vi "PelletronQuery.vi"() -> ()   [LabVIEW 2012]
uses:
  <vilib>/Utility/miscctls.llb/LVPointTypeDef.ctl
  <vilib>/addons/database/Auxilliary.llb/DB Tools Cursor Type.ctl
  <userlib>/_OpenG.lib/array/array.llb/Index 1D Array Elements (String)__ogtk.vi
  <vilib>/addons/database/Connection.llb/Conn Execute.vi
  <vilib>/addons/database/Recordset.llb/Rec Fetch Recordset Data (R).vi
  <vilib>/addons/database/Recordset.llb/Rec Destroy - Connection.vi
  <vilib>/Utility/file.llb/Write To Spreadsheet File (string).vi
  <vilib>/addons/database/_DB Variant To Data/Database Variant To Data.xnode
  <vilib>/addons/database/NI_Database_API.lvlib
panel:
  in  "stop":bool
  in  "Tab Control":T1(tab)
  in  "Active Y Scale":u16(ring) items=["Voltage (MV)", "Current (µA)", "Voltage (kV)", "Pressure (torr)", "Radiation (mr/hr)"]
  in  "X Maximum":dbl format="%<%I:%M:%S %p\n%m/%d/%Y>T"
  in  "X Autoscale":bool=TRUE
  in  "X Minimum":dbl format="%<%I:%M:%S %p\n%m/%d/%Y>T"
  in  "Y Autoscale":bool=TRUE
  in  "Y Maximum":dbl
  in  "Y Minimum":dbl
  in  "Plot":bool
  in  "Limits":T2={"Lower Timestamp Range"=timestamp(0 s since 1904-01-01), "Upper Timestamp Range"=timestamp(0 s since 1904-01-01), "Lower High Voltage"=0.0, "Higher High Voltage"=inf, "Lower Power Supply"=0.0, "Higher Power Supply"=inf}
  in  "Independent Variable":enum32{"Time", "ID"}(radio)
  in  "Pelletron Properties":i32[](listbox)
  out "XY Graph":cluster{ext[], dbl[]}[](graph)
  in  "Write":bool
  in  "Pull Data":bool
  in  "Limits 2":T2
  out "Pelletron Data":string[][](table)
  in  "Save Path":path=path "C:/Users/Clavius/Desktop/Database Query files/New_Pelletron_Query.csv"
  out "error out":errorcluster
  in  "Clear Errors?":bool
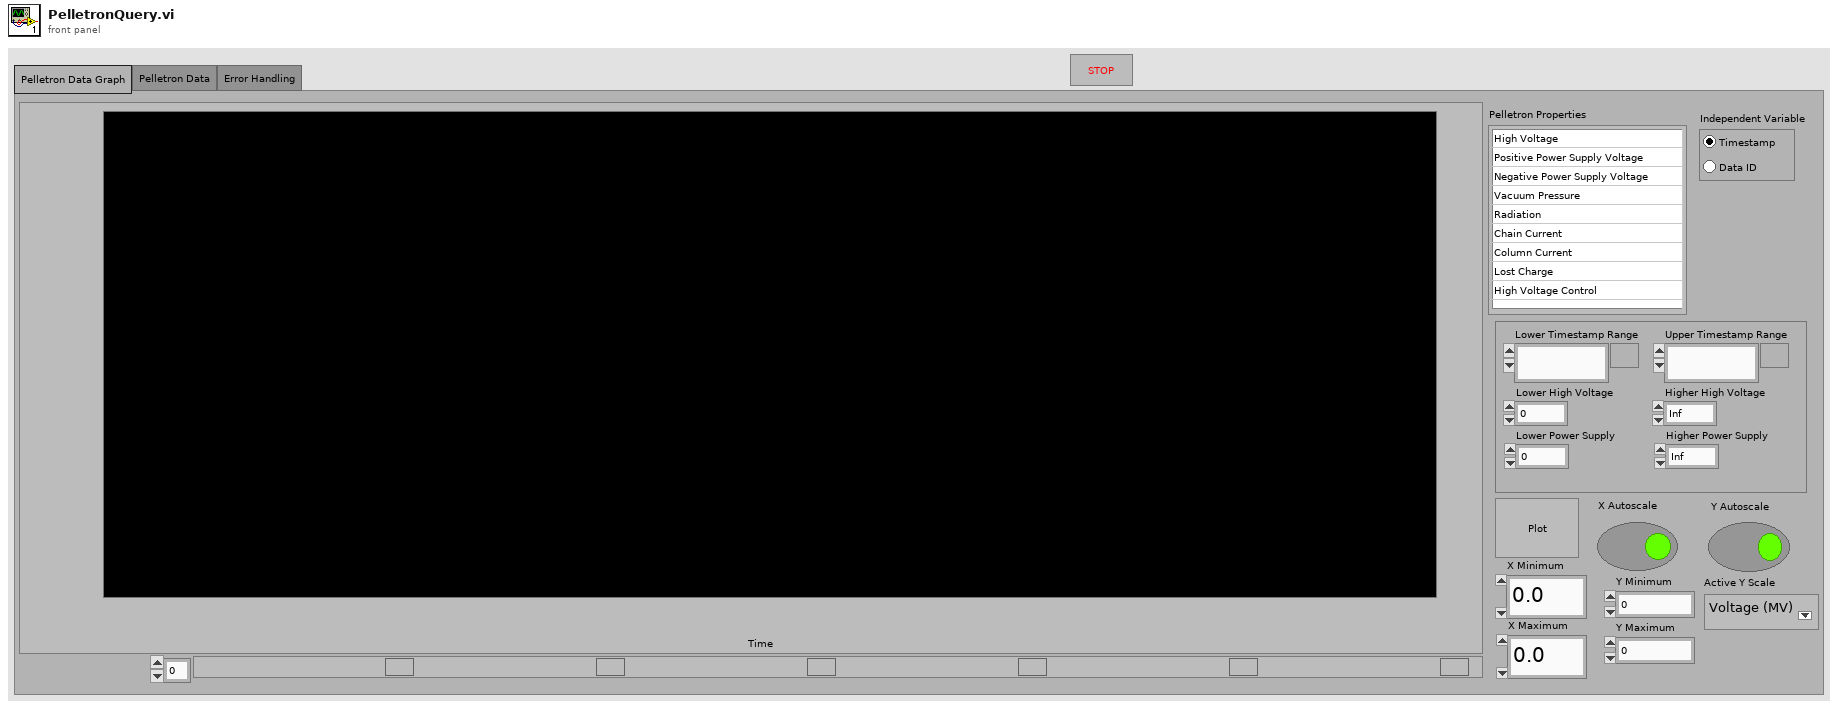
[diagram p1: front panel]
types:
  T1 = enum32{"Pelletron Data Graph", "Pelletron Data", "Error Handling"}
  T2 = cluster{"Lower Timestamp Range":timestamp, "Upper Timestamp Range":timestamp, "Lower High Voltage":dbl, "Higher High Voltage":dbl, "Lower Power Supply":dbl, "Higher Power Supply":dbl}
  T3 = typedef "LVPointTypeDef.ctl" = cluster{"Horizontal":i16, "Vertical":i16}
  T4 = typedef "NI_Database_API.lvlib/DB Tools Cursor Type.ctl" = enum16{"forward-only", "keyset", "dynamic", "static"}
  T5 = cluster{"Pelletron ID":i32[], "Integer Timestamp":dbl[], "High Voltage":dbl[], "Positive High Voltage Supply":dbl[], "Negative High Voltage Supply":dbl[], "Vaccuum Pressure":dbl[], "Radiation":dbl[], "Chain Current":dbl[], "Column Current":dbl[], "Lost Charge":dbl[], "High Voltage Control":dbl[], "Control Difference":dbl[]}
  T6 = typedef "NI_Database_API.lvlib/Conn ObjectReference.ctl" = refnum<k1>
  T7 = typedef "NI_Database_API.lvlib/Rec ObjectReference.ctl" = refnum<k1>
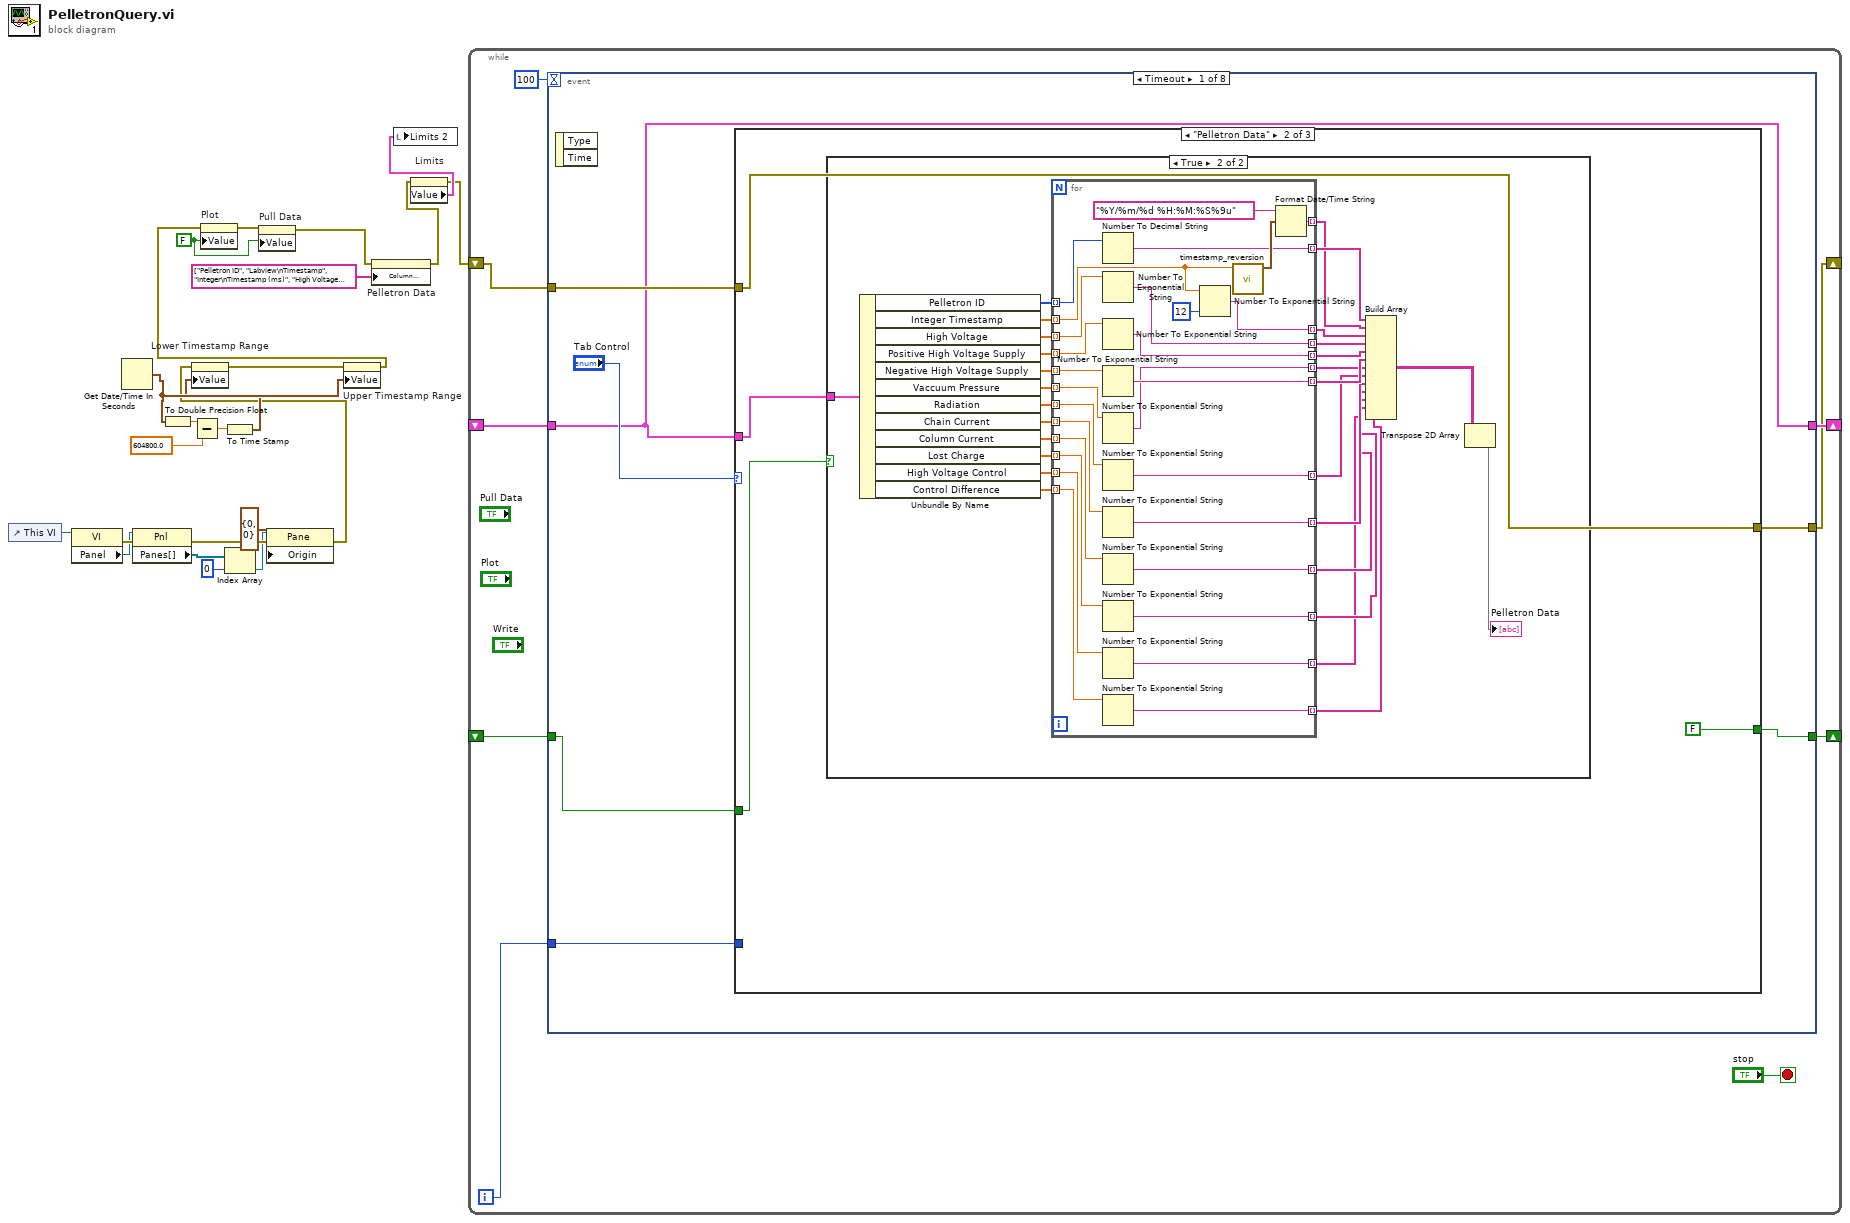
[diagram p0: block diagram]
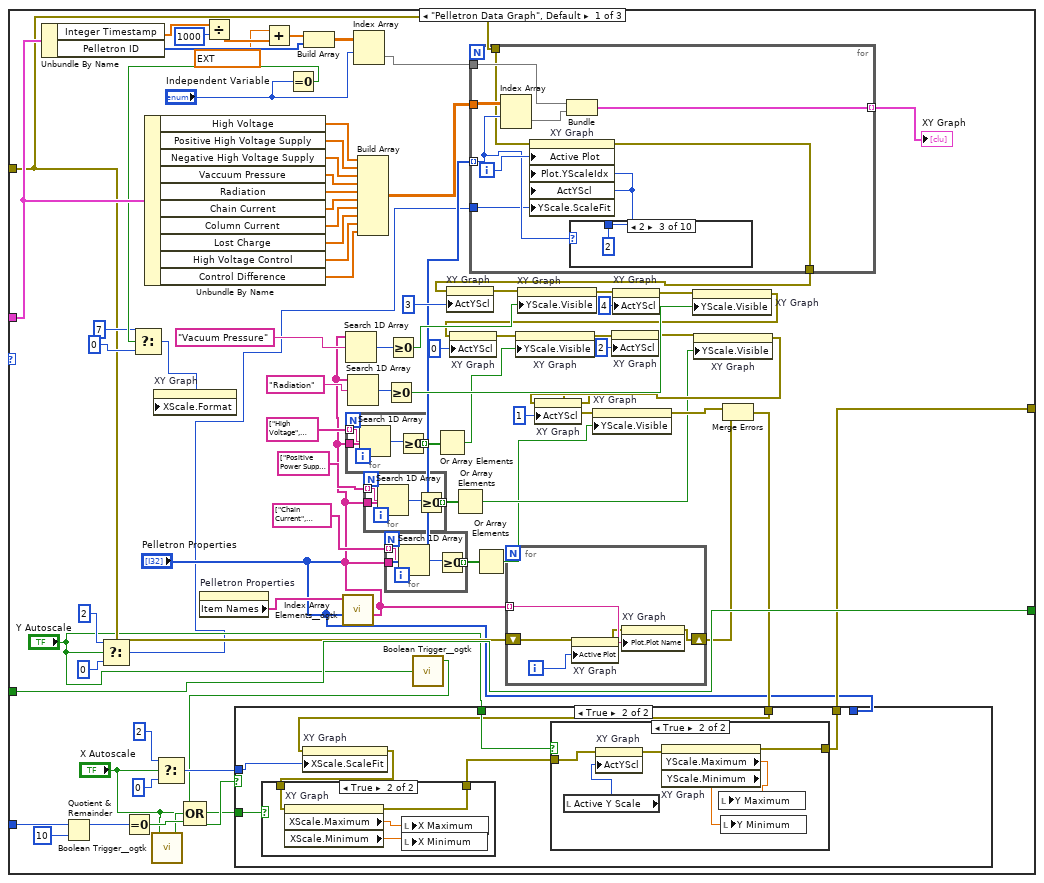
[diagram p2: hidden frame]
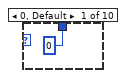
[diagram p6: hidden frame]
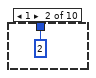
[diagram p7: hidden frame]
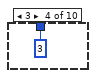
[diagram p8: hidden frame]
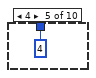
[diagram p9: hidden frame]
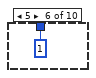
[diagram p10: hidden frame]
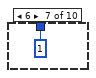
[diagram p11: hidden frame]
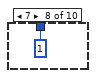
[diagram p12: hidden frame]
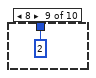
[diagram p13: hidden frame]
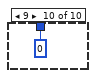
[diagram p14: hidden frame]
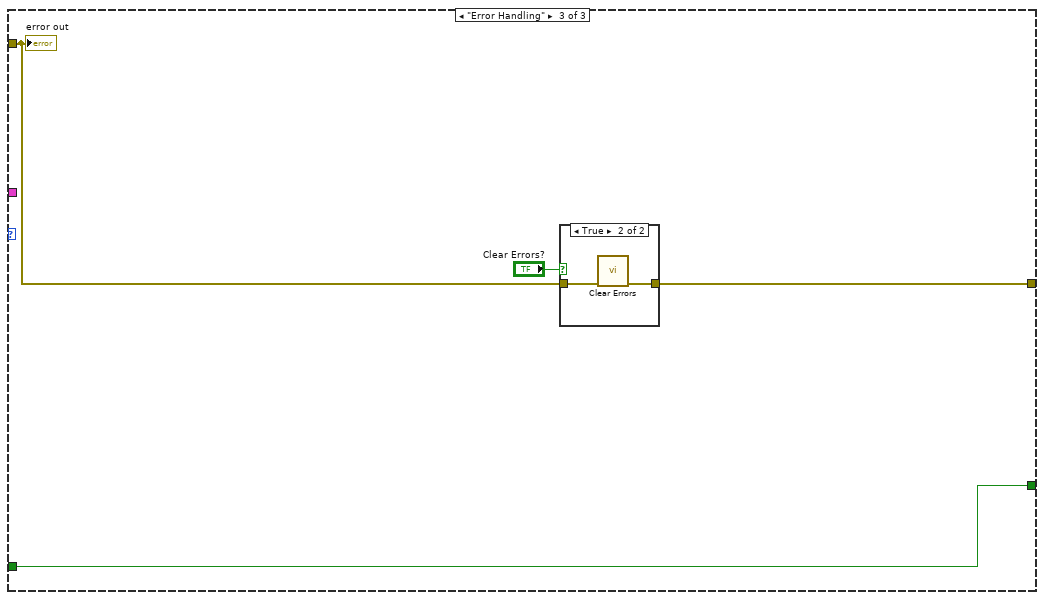
[diagram p16: hidden frame]
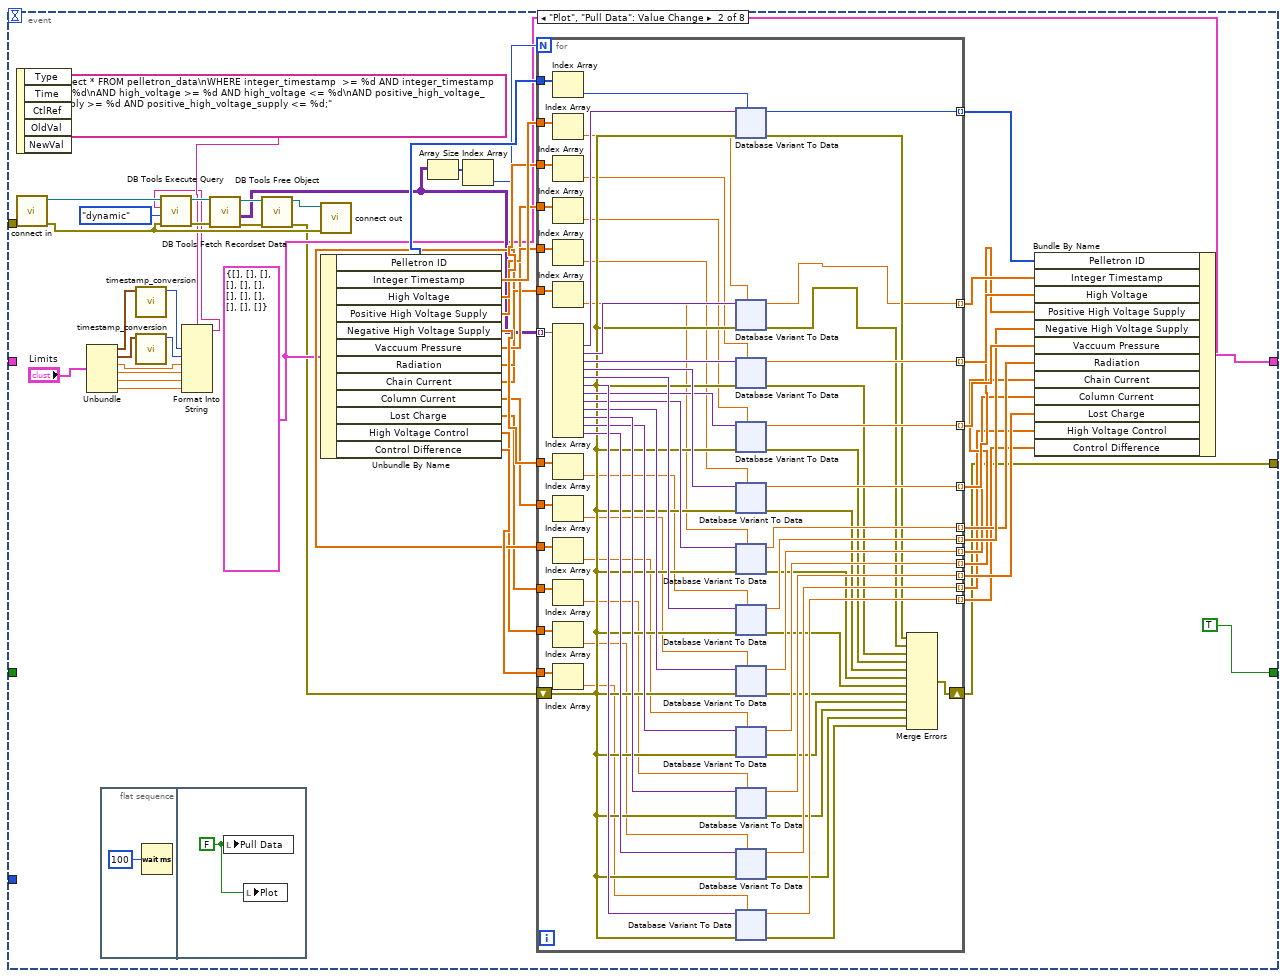
[diagram p18: hidden frame]
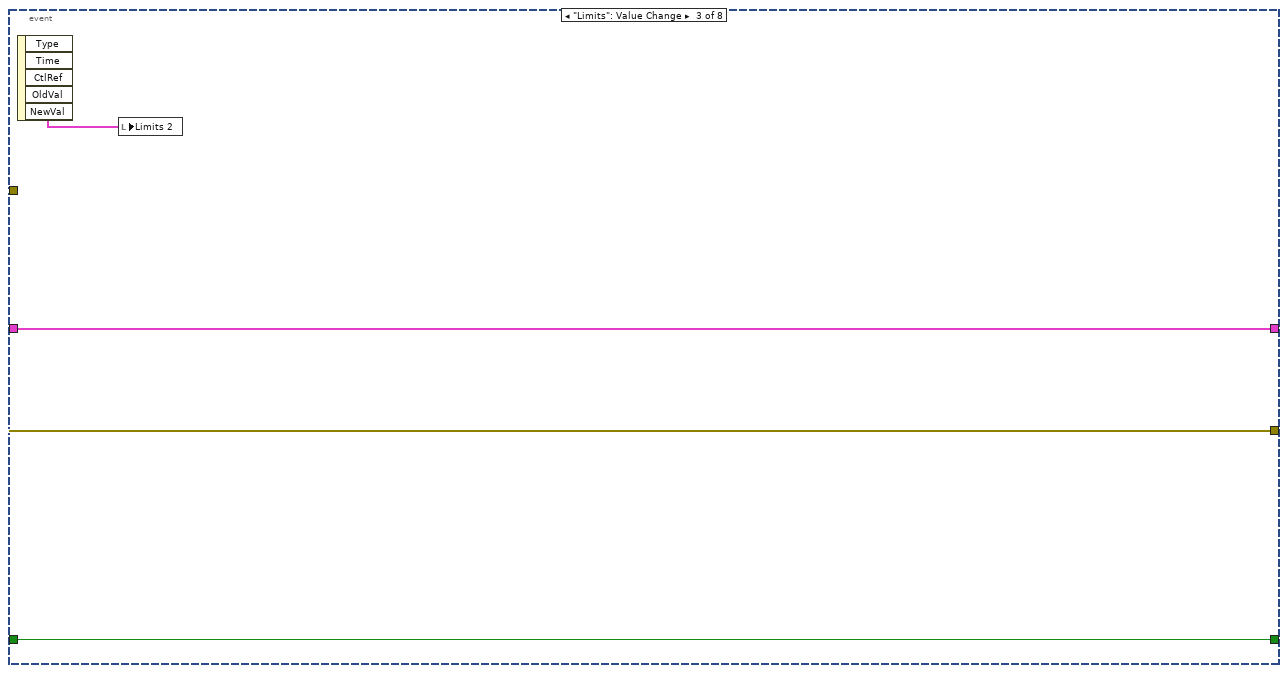
[diagram p19: hidden frame]
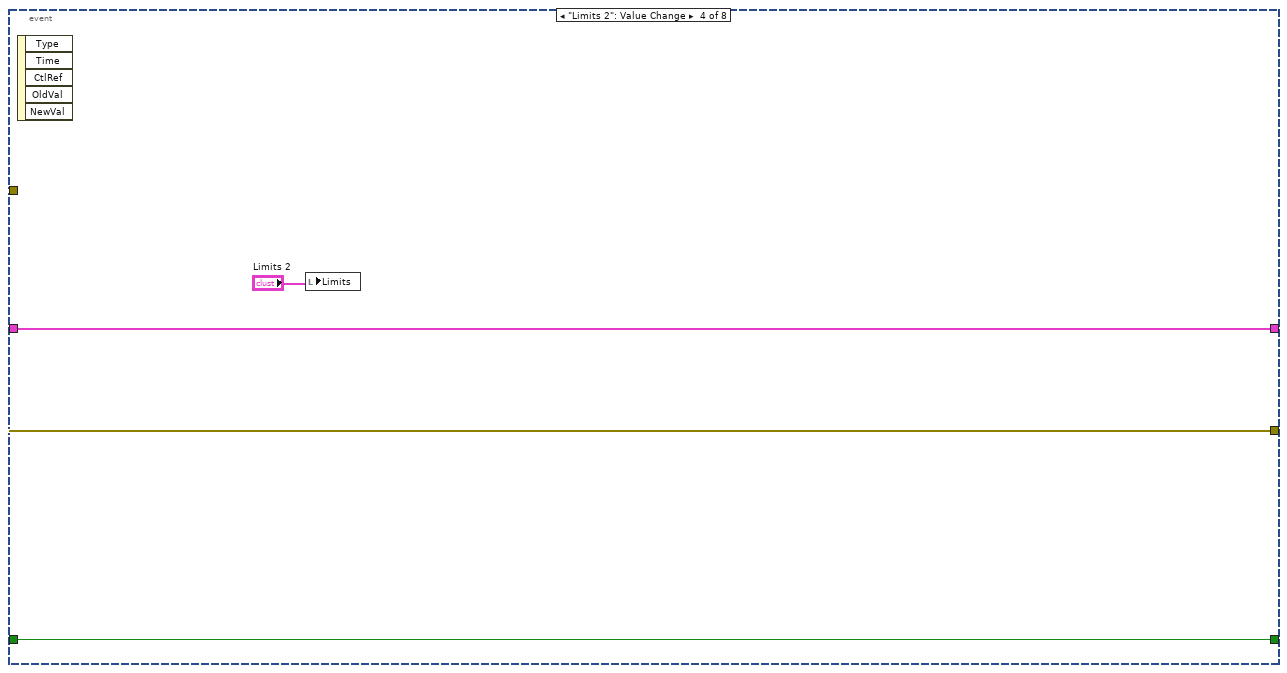
[diagram p20: hidden frame]
diagram:
  w20 = FALSE ("Plot")
  n1 = control-ref of="This VI"() -> (w9:refnum<vi>)
  n2 = property class="VI"(reference=w9) -> (error out=w8:errorcluster, "Panel"=w7:refnum<vi>)  [unwired: 1 in, 1 out]
  n3 = Get Date/Time In Seconds() -> (seconds since 1Jan1904=w17:timestamp)
  n4 = property class="Pnl"(reference=w7, error in=w8) -> (error out=w6:errorcluster, "Panes[]"=w5:refnum<vi>[])  [unwired: 1 out]
  n5 = To Double Precision Float(number=w17) -> (double precision float=w16:dbl)
  n6 = Subtract(x=w16, y=604800.0) -> (x-y=w14:dbl)
  n7 = To Time Stamp(1:w14) -> (0:w13:timestamp)
  n8 = Index Array(array=w5, index=0) -> (element=w3:refnum<vi>)
  n9 = property class="Pane"(reference=w3, error in=w6, "Origin"=T3 {"Horizontal"=0, "Vertical"=0}) -> (error out=w1:errorcluster)  [unwired: 1 out]
  n10 = property on="Lower Timestamp Range" class="AbsTime (strict)"(error in=w1, "Value"=w13) -> (error out=w19:errorcluster)  [unwired: 1 in, 1 out]
  n11 = property on="Upper Timestamp Range" class="AbsTime (strict)"(error in=w19, "Value"=w17) -> (error out=w18:errorcluster)  [unwired: 1 in, 1 out]
  n12 = property on="Plot" class="Bool (strict)"(error in=w18, "Value"=w20) -> (error out=w22:errorcluster)  [unwired: 1 in, 1 out]
  n13 = property on="Pull Data" class="Bool (strict)"(error in=w22, "Value"=w20) -> (error out=w21:errorcluster)  [unwired: 1 in, 1 out]
  n14 = property on="Pelletron Data" class="Tbl (strict)"(error in=w21, "Column Headers[]"=string[] ["Pelletron ID", "Labview\nTimestamp", "Integer\nTimestamp (ms)", "High Voltage (MV)", "Positive Power\nSupply Voltage (kV)", "Negative Power\nSupply Voltage (kV)", "Vacuum\nPressure (Torr)", "Radiation\n(mrad/hr)", "Chain\nCurrent (µA)", "Column\nCurrent (µA)", "Lost\nCharge (µA)", "High Voltage\nControl (MV)", "Control\nDifference (kV)"]) -> (error out=w11:errorcluster)  [unwired: 1 in, 1 out]
  n15 = property on="Limits" class="Clust (strict)"(error in=w11) -> (error out=w10:errorcluster, "Value"=w12:T2)  [unwired: 1 in, 1 out]
  n16 = local write "Limits 2"(w12) -> ()
  n17 = while {
    shift-right: [w29] -> _
    shift-left: w10 -> [w31]
    shift-right: [w30] -> _
    shift-left: _ -> [w28]
    shift-right: [w26] -> _
    shift-left: _ -> [w25]
    i -> [w24]
    stop <- "stop" stop-if-true
    n18 = event shown="[0] Timeout" {
      selector: _ -> [_ _ _ _ _ _ _ _]
      dyn-events: _ -> [_ _ _ _ _ _ _ _]
      timeout: 100 -> [_ _ _ _ _ _ _ _]
      tunnel: w31 -> [w38 w293 w747 w751 w756 w766 w776 w782]
      tunnel: w28 -> [w36 _ w746 w750 w754 w764 w775 w783]
      tunnel: [w36 w259 w746 w750 w754 w764 w775 w783] -> w30
      tunnel: [w37 w245 w747 w751 w755 w765 w776 w782] -> w29
      tunnel: [w35 TRUE w745 w749 w753 w763 w774 w781] -> w26
      tunnel: w25 -> [w34 _ w745 w749 w753 w763 w774 w781]
      tunnel: w24 -> [w33 _ _ _ _ _ _ _]
      event Timeout {
        n19 = event-data() -> ()  [unwired: 1 in, 2 out]
        n20 = case shown="\"Pelletron Data\"" "Tab Control" {
          tunnel: w38 -> [w60 w179 w240]
          tunnel: [w58 w179 w239] -> w37
          tunnel: w36 -> [w119 w180 _]
          tunnel: [w118 FALSE w237] -> w35
          tunnel: w34 -> [w118 w177 w237]
          tunnel: w33 -> [w57 _ _]
          frame "Pelletron Data Graph", Default {
            n21 = Unbundle By Name(w119) -> ("Integer Timestamp"=w43:dbl[], "Pelletron ID"=w117:i32[])
            n22 = Quotient & Remainder(x=w57, y=10) -> (x-y*floor(x/y)=w54:i32)  [unwired: 1 out]
            n23 = Select(t=u8 2 ("X Scale.Scale Fit"), s="Y Autoscale", f=u8 0 ("X Scale.Scale Fit")) -> (s? t:f=w46:u8)
            n24 = Equal To 0?(x=w54) -> (x = 0?=w53:bool)
            n25 = Unbundle By Name(w119) -> ("High Voltage"=w115:dbl[], "Positive High Voltage Supply"=w114:dbl[], "Negative High Voltage Supply"=w113:dbl[], "Vaccuum Pressure"=w70:dbl[], "Radiation"=w71:dbl[], "Chain Current"=w112:dbl[], "Column Current"=w111:dbl[], "Lost Charge"=w110:dbl[], "High Voltage Control"=w109:dbl[], "Control Difference"=w108:dbl[])
            n26 = call <userlib>:"Boolean Trigger__ogtk.vi"("Boolean Input"="X Autoscale") -> ("Rising Edge"=w51:bool)  [unwired: 1 in, 1 out]
            n27 = Select(t=u8 2 ("X Scale.Scale Fit"), s="X Autoscale", f=u8 0 ("X Scale.Scale Fit")) -> (s? t:f=w68:u8)
            n28 = property on="Pelletron Properties" class="LstBox (strict)"() -> ("Item Names"=w104:string[])  [unwired: 2 in, 2 out]
            n29 = Divide(x=w43, y=1000) -> (x/y=w44:dbl[])
            n30 = Add(x=ext 2082844800.0, y=w44) -> (x+y=w41:ext[])
            n31 = Equal To 0?(x="Independent Variable") -> (x = 0?=w64:bool)
            n32 = Select(t=u8 7 ("X Scale.Display Format:Format"), s=w64, f=u8 0 ("X Scale.Display Format:Format")) -> (s? t:f=w61:u8)
            n33 = property on="XY Graph" class="XYGraph (strict)"("XScale.Format"=w61) -> ()  [unwired: 2 in, 2 out]
            n34 = Build Array(w41, w117) -> (w116:ext[][])
            n35 = call-poly <userlib>:"Index Array Elements__ogtk.vi"("indices"="Pelletron Properties", "array"=w104) -> ("elements"=w74:string[])  [unwired: 9 in]
            n36 = Search 1D Array(1D array=w74, element="Vacuum Pressure") -> (index of element=w100:i32)  [unwired: 1 in]
            n37 = for {
              tunnel: string[] ["High Voltage", "High Voltage Control"] -> [w150] mode=indexing
              tunnel: w74 -> [w149]
              tunnel: [w148] -> w80 mode=indexing
              n38 = Search 1D Array(1D array=w149, element=w150) -> (index of element=w151:i32)  [unwired: 1 in]
              n39 = Greater Or Equal To 0?(x=w151) -> (x >= 0?=w148:bool)
            }
            n40 = Search 1D Array(1D array=w74, element="Radiation") -> (index of element=w99:i32)  [unwired: 1 in]
            n41 = Index Array(array=w116, index (row)="Independent Variable") -> (element=w106:ext[])  [unwired: 1 in]
            n42 = Build Array(w115, w114, w113, w70, w71, w112, w111, w110, w109, w108) -> (w107:dbl[][])
            n43 = for {
              tunnel: string[] ["Positive Power Supply Voltage", "Negative Power Supply Voltage", "Control Difference"] -> [w146] mode=indexing
              tunnel: w74 -> [w145]
              tunnel: [w144] -> w76 mode=indexing
              n44 = Search 1D Array(1D array=w145, element=w146) -> (index of element=w147:i32)  [unwired: 1 in]
              n45 = Greater Or Equal To 0?(x=w147) -> (x >= 0?=w144:bool)
            }
            n46 = for {
              tunnel: string[] ["Chain Current", "Column Current", "Lost Charge"] -> [w142] mode=indexing
              tunnel: w74 -> [w141]
              tunnel: [w140] -> w73 mode=indexing
              n47 = Search 1D Array(1D array=w141, element=w142) -> (index of element=w143:i32)  [unwired: 1 in]
              n48 = Greater Or Equal To 0?(x=w143) -> (x >= 0?=w140:bool)
            }
            n49 = Greater Or Equal To 0?(x=w99) -> (x >= 0?=w92:bool)
            n50 = Greater Or Equal To 0?(x=w100) -> (x >= 0?=w96:bool)
            n51 = call <userlib>:"Boolean Trigger__ogtk.vi"("Boolean Input"="Y Autoscale") -> ("Rising Edge"=w48:bool)  [unwired: 1 in, 1 out]
            n52 = Compound Arithmetic op=OR(w48, w51, w53) -> (w52:bool)
            n53 = Or Array Elements(Boolean array=w80) -> (logical OR=w79:bool)
            n54 = Or Array Elements(Boolean array=w76) -> (logical OR=w77:bool)
            n55 = for {
              tunnel: "Pelletron Properties" -> [w161] mode=indexing
              tunnel: w107 -> [w166]
              tunnel: w106 -> [w165]
              tunnel: [w163] -> w105 mode=indexing
              tunnel: w60 -> [w160]
              tunnel: [w159] -> w45
              tunnel: w46 -> [w157]
              i -> [w162]
              n56 = Index Array(array=w166, index (row)=w161) -> (element=w164:dbl[])  [unwired: 1 in]
              n57 = Bundle(w165, w164) -> (w163:cluster{ext[], dbl[]})  [unwired: 1 in]
              n58 = case shown="2" w161 {
                tunnel: [u32 0 ("Plot.Y Scale Index") u32 2 ("Plot.Y Scale Index") u32 2 ("Plot.Y Scale Index") u32 3 ("Plot.Y Scale Index") u32 4 ("Plot.Y Scale Index") u32 1 ("Plot.Y Scale Index") u32 1 ("Plot.Y Scale Index") u32 1 ("Plot.Y Scale Index") u32 2 ("Plot.Y Scale Index") u32 0 ("Plot.Y Scale Index")] -> w158
                frame 0, Default {
                }
                frame 1 {
                }
                frame 2 {
                }
                frame 3 {
                }
                frame 4 {
                }
                frame 5 {
                }
                frame 6 {
                }
                frame 7 {
                }
                frame 8 {
                }
                frame 9 {
                }
              }
              n59 = property on="XY Graph" class="XYGraph (strict)"(error in=w160, "Active Plot"=w162, "Plot.YScaleIdx"=w158, "ActYScl"=w158, "YScale.ScaleFit"=w157) -> (error out=w159:errorcluster)  [unwired: 1 in, 1 out]
            }
            "XY Graph" <- w105
            n60 = property on="XY Graph" class="XYGraph (strict)"(error in=w45, "ActYScl"=3 ("Active Y Scale")) -> (error out=w97:errorcluster)  [unwired: 1 in, 1 out]
            n61 = Or Array Elements(Boolean array=w73) -> (logical OR=w72:bool)
            n62 = for {
              tunnel: w74 -> [w155] mode=indexing
              shift-right: [w153] -> w103
              shift-left: w60 -> [w152]
              i -> [w156]
              n63 = property on="XY Graph" class="XYGraph (strict)"(error in=w152, "Active Plot"=w156) -> (error out=w154:errorcluster)  [unwired: 1 in, 1 out]
              n64 = property on="XY Graph" class="XYGraph (strict)"(error in=w154, "Plot.Plot Name"=w155) -> (error out=w153:errorcluster)  [unwired: 1 in, 1 out]
            }
            n65 = property on="XY Graph" class="XYGraph (strict)"(error in=w97, "YScale.Visible"=w96) -> (error out=w95:errorcluster)  [unwired: 1 in, 1 out]
            n66 = property on="XY Graph" class="XYGraph (strict)"(error in=w95, "ActYScl"=4 ("Active Y Scale")) -> (error out=w93:errorcluster)  [unwired: 1 in, 1 out]
            n67 = property on="XY Graph" class="XYGraph (strict)"(error in=w93, "YScale.Visible"=w92) -> (error out=w91:errorcluster)  [unwired: 1 in, 1 out]
            n68 = property on="XY Graph" class="XYGraph (strict)"(error in=w91, "ActYScl"=0 ("Active Y Scale")) -> (error out=w89:errorcluster)  [unwired: 1 in, 1 out]
            n69 = property on="XY Graph" class="XYGraph (strict)"(error in=w89, "YScale.Visible"=w79) -> (error out=w88:errorcluster)  [unwired: 1 in, 1 out]
            n70 = property on="XY Graph" class="XYGraph (strict)"(error in=w88, "ActYScl"=2 ("Active Y Scale")) -> (error out=w86:errorcluster)  [unwired: 1 in, 1 out]
            n71 = property on="XY Graph" class="XYGraph (strict)"(error in=w86, "YScale.Visible"=w77) -> (error out=w85:errorcluster)  [unwired: 1 in, 1 out]
            n72 = property on="XY Graph" class="XYGraph (strict)"(error in=w85, "ActYScl"=1 ("Active Y Scale")) -> (error out=w83:errorcluster)  [unwired: 1 in, 1 out]
            n73 = property on="XY Graph" class="XYGraph (strict)"(error in=w83, "YScale.Visible"=w72) -> (error out=w82:errorcluster)  [unwired: 1 in, 1 out]
            n74 = Merge Errors(w82, w103) -> (w59:errorcluster)
            n75 = case shown="True" w52 {
              tunnel: w68 -> [_ w127]
              tunnel: "Y Autoscale" -> [_ w126]
              tunnel: w59 -> [w120 w123]
              tunnel: [w120 w121] -> w58
              tunnel: "X Autoscale" -> [_ w122]
              tunnel: "Pelletron Properties" -> [_ _]
              frame False {
              }
              frame True {
                n76 = property on="XY Graph" class="XYGraph (strict)"(error in=w123, "XScale.ScaleFit"=w127) -> (error out=w125:errorcluster)  [unwired: 1 in, 1 out]
                n77 = case shown="True" w122 {
                  tunnel: w125 -> [w135 w137]
                  tunnel: [w135 w136] -> w124
                  frame False {
                  }
                  frame True {
                    n78 = property on="XY Graph" class="XYGraph (strict)"(error in=w137) -> (error out=w136:errorcluster, "XScale.Maximum"=w139:dbl, "XScale.Minimum"=w138:dbl)  [unwired: 1 in, 1 out]
                    n79 = local write "X Maximum"(w139) -> ()
                    n80 = local write "X Minimum"(w138) -> ()
                  }
                }
                n81 = case shown="True" w126 {
                  tunnel: w124 -> [w128 w130]
                  tunnel: [w128 w129] -> w121
                  frame False {
                  }
                  frame True {
                    n82 = local read "Active Y Scale"() -> (w133:u16)
                    n83 = property on="XY Graph" class="XYGraph (strict)"(error in=w130, "ActYScl"=w133) -> (error out=w134:errorcluster)  [unwired: 1 in, 1 out]
                    n84 = property on="XY Graph" class="XYGraph (strict)"(error in=w134) -> (error out=w129:errorcluster, "YScale.Maximum"=w132:dbl, "YScale.Minimum"=w131:dbl)  [unwired: 1 in, 1 out]
                    n85 = local write "Y Maximum"(w132) -> ()
                    n86 = local write "Y Minimum"(w131) -> ()
                  }
                }
              }
            }
          }
          frame "Pelletron Data" {
            n87 = case shown="True" w177 {
              tunnel: w180 -> [_ w208]
              frame False {
              }
              frame True {
                n88 = Unbundle By Name(w208) -> ("Pelletron ID"=w207:i32[], "Integer Timestamp"=w206:dbl[], "High Voltage"=w205:dbl[], "Positive High Voltage Supply"=w204:dbl[], "Negative High Voltage Supply"=w203:dbl[], "Vaccuum Pressure"=w202:dbl[], "Radiation"=w201:dbl[], "Chain Current"=w200:dbl[], "Column Current"=w199:dbl[], "Lost Charge"=w198:dbl[], "High Voltage Control"=w197:dbl[], "Control Difference"=w196:dbl[])
                n89 = for {
                  tunnel: w207 -> [w234] mode=indexing
                  tunnel: w206 -> [w211] mode=indexing
                  tunnel: w205 -> [w233] mode=indexing
                  tunnel: w204 -> [w232] mode=indexing
                  tunnel: w203 -> [w231] mode=indexing
                  tunnel: w202 -> [w230] mode=indexing
                  tunnel: w201 -> [w229] mode=indexing
                  tunnel: w200 -> [w228] mode=indexing
                  tunnel: w199 -> [w227] mode=indexing
                  tunnel: w198 -> [w226] mode=indexing
                  tunnel: w197 -> [w225] mode=indexing
                  tunnel: w196 -> [w224] mode=indexing
                  tunnel: [w223] -> w183 mode=indexing
                  tunnel: [w222] -> w182 mode=indexing
                  tunnel: [w221] -> w195 mode=indexing
                  tunnel: [w220] -> w194 mode=indexing
                  tunnel: [w219] -> w193 mode=indexing
                  tunnel: [w218] -> w192 mode=indexing
                  tunnel: [w217] -> w191 mode=indexing
                  tunnel: [w216] -> w190 mode=indexing
                  tunnel: [w215] -> w189 mode=indexing
                  tunnel: [w214] -> w188 mode=indexing
                  tunnel: [w213] -> w187 mode=indexing
                  tunnel: [w212] -> w186 mode=indexing
                  tunnel: [w209] -> w181 mode=indexing
                  n90 = Number To Decimal String(number=w234) -> (decimal integer string=w223:string)  [unwired: 1 in]
                  n91 = Number To Exponential String(number=w233) -> (E-format string=w221:string)  [unwired: 3 in]
                  n92 = Number To Exponential String(number=w232) -> (E-format string=w220:string)  [unwired: 3 in]
                  n93 = Number To Exponential String(number=w231) -> (E-format string=w219:string)  [unwired: 3 in]
                  n94 = Number To Exponential String(number=w230) -> (E-format string=w218:string)  [unwired: 3 in]
                  n95 = Number To Exponential String(number=w229) -> (E-format string=w217:string)  [unwired: 3 in]
                  n96 = Number To Exponential String(number=w228) -> (E-format string=w216:string)  [unwired: 3 in]
                  n97 = Number To Exponential String(number=w227) -> (E-format string=w215:string)  [unwired: 3 in]
                  n98 = Number To Exponential String(number=w226) -> (E-format string=w214:string)  [unwired: 3 in]
                  n99 = Number To Exponential String(number=w225) -> (E-format string=w213:string)  [unwired: 3 in]
                  n100 = Number To Exponential String(number=w224) -> (E-format string=w212:string)  [unwired: 3 in]
                  n101 = Number To Exponential String(number=w211, precision (6)=i16 12) -> (E-format string=w209:string)  [unwired: 2 in]
                  n102 = call "timestamp_reversion.vi"("Integer Timestamp"=w211) -> ("time stamp"=w235:timestamp)  [unwired: 8 in, 1 out]
                  n103 = Format Date/Time String(time format string (%c)="%Y/%m/%d %H:%M:%S%9u", seconds (now)=w235) -> (date/time string=w222:string)  [unwired: 1 in]
                }
                n104 = Build Array(w183, w182, w181, w195, w194, w193, w192, w191, w190, w189, w188, w187, w186) -> (w185:string[][])
                n105 = Transpose 2D Array(2D array=w185) -> (transposed array=→"Pelletron Data":string[][])
              }
            }
          }
          frame "Error Handling" {
            n106 = case shown="True" "Clear Errors?" {
              tunnel: w240 -> [w241 w243]
              tunnel: [w241 w242] -> w239
              frame False {
              }
              frame True {
                n107 = call <vilib>:"Clear Errors.vi"("error in (no error)"=w243) -> ("error out"=w242:errorcluster)  [unwired: 6 in]
              }
            }
            "error out" <- w240
          }
        }
      }
      event "Plot", "Pull Data": Value Change {
        w258 = T5 {"Pelletron ID"=[], "Integer Timestamp"=[], "High Voltage"=[], "Positive High Voltage Supply"=[], "Negative High Voltage Supply"=[], "Vaccuum Pressure"=[], "Radiation"=[], "Chain Current"=[], "Column Current"=[], "Lost Charge"=[], "High Voltage Control"=[], "Control Difference"=[]} ("Cluster")
        n108 = event-data() -> ()  [unwired: 1 in, 5 out]
        n109 = call "connect in.vi"("error in (no error)"=w293) -> ("error out"=w290:errorcluster, "Database Connection"=w294:T6)  [unwired: 6 in, 1 out]
        n110 = Unbundle("Limits") -> ("Lower Timestamp Range"=w254:timestamp, "Upper Timestamp Range"=w253:timestamp, "Lower High Voltage"=w250:dbl, "Higher High Voltage"=w249:dbl, "Lower Power Supply"=w248:dbl, "Higher Power Supply"=w247:dbl)
        n111 = flat-sequence {
          frame #0 {
            n112 = Wait (ms)(milliseconds to wait=u32 100) -> ()  [unwired: 1 out]
          }
          frame #1 {
            w297 = FALSE ("Pull Data")
            n113 = local write "Pull Data"(w297) -> ()
            n114 = local write "Plot"(w297) -> ()
          }
        }
        n115 = call "timestamp_conversion.vi"("Time Stamp"=w254) -> ("Integer Time"=w252:i64)  [unwired: 8 in, 1 out]
        n116 = call "timestamp_conversion.vi"("Time Stamp"=w253) -> ("Integer Time"=w251:i64)  [unwired: 8 in, 1 out]
        n117 = Format Into String(format string="Select * FROM pelletron_data\nWHERE integer_timestamp  >= %d AND integer_timestamp <= %d\nAND high_voltage >= %d AND high_voltage <= %d\nAND positive_high_voltage_supply >= %d AND positive_high_voltage_supply <= %d;", w252, w251, w250, w249, w248, w247) -> (resulting string=w256:string)  [unwired: 2 in, 1 out]
        n118 = call-poly <vilib>:"DB Tools Execute Query.vi"("error in (no error)"=w290, "cursor type"=DB_Tools_Cursor_Type."dynamic", "SQL query"=w256, "connection reference"=w294) -> ("error out"=w291:errorcluster, "recordset reference"=w289:T7)  [unwired: 4 in]
        n119 = call-poly <vilib>:"DB Tools Fetch Recordset Data.vi"("error in (no error)"=w291, "recordset reference"=w289) -> ("error out"=w292:errorcluster, "recordset data"=w274:variant[][], "recordset reference out"=w288:T7)  [unwired: 3 in]
        n120 = call-poly <vilib>:"DB Tools Free Object.vi"("error in (no error)"=w292, "recordset reference"=w288) -> ("error out"=w246:errorcluster, "connection reference"=w287:T6)  [unwired: 8 in]
        n121 = call "connect out.vi"("error in (no error)"=w290, "connection reference"=w287) -> ()  [unwired: 9 in, 1 out]
        n122 = Unbundle By Name(w258) -> ("Pelletron ID"=w286:i32[], "Integer Timestamp"=w285:dbl[], "High Voltage"=w284:dbl[], "Positive High Voltage Supply"=w283:dbl[], "Negative High Voltage Supply"=w282:dbl[], "Vaccuum Pressure"=w280:dbl[], "Radiation"=w279:dbl[], "Chain Current"=w278:dbl[], "Column Current"=w277:dbl[], "Lost Charge"=w276:dbl[], "High Voltage Control"=w275:dbl[], "Control Difference"=w281:dbl[])
        n123 = Array Size(array=w274) -> (size(s)=w273:i32[])
        n124 = Index Array(array=w273) -> (element=w272:i32)  [unwired: 1 in]
        n125 = for {
          N: w272 -> [_]
          tunnel: w274 -> [w360] mode=indexing
          tunnel: w286 -> [w347]
          tunnel: w285 -> [w346]
          tunnel: w284 -> [w345]
          tunnel: w283 -> [w344]
          tunnel: w282 -> [w343]
          tunnel: w281 -> [w342]
          tunnel: w280 -> [w341]
          tunnel: w279 -> [w340]
          tunnel: w278 -> [w339]
          tunnel: w277 -> [w338]
          tunnel: w276 -> [w337]
          tunnel: w275 -> [w336]
          tunnel: [w335] -> w271 mode=indexing
          tunnel: [w299] -> w270 mode=indexing
          tunnel: [w334] -> w269 mode=indexing
          tunnel: [w333] -> w268 mode=indexing
          tunnel: [w332] -> w267 mode=indexing
          tunnel: [w331] -> w266 mode=indexing
          tunnel: [w330] -> w265 mode=indexing
          tunnel: [w329] -> w264 mode=indexing
          tunnel: [w328] -> w263 mode=indexing
          tunnel: [w327] -> w262 mode=indexing
          tunnel: [w326] -> w261 mode=indexing
          tunnel: [w325] -> w260 mode=indexing
          shift-right: [w312] -> w245
          shift-left: w246 -> [w324]
          n126 = Index Array(array=w347) -> (element=w311:i32)  [unwired: 1 in]
          n127 = Index Array(array=w346) -> (element=w310:dbl)  [unwired: 1 in]
          n128 = Index Array(array=w345) -> (element=w309:dbl)  [unwired: 1 in]
          n129 = Index Array(array=w341) -> (element=w305:dbl)  [unwired: 1 in]
          n130 = Index Array(array=w344) -> (element=w308:dbl)  [unwired: 1 in]
          n131 = Index Array(array=w340) -> (element=w304:dbl)  [unwired: 1 in]
          n132 = Index Array(array=w360) -> (element #1=w359:variant, element #2=w358:variant, element #3=w357:variant, element #4=w356:variant, element #5=w355:variant, element #6=w354:variant, element #7=w353:variant, element #8=w352:variant, element #9=w351:variant, element #10=w350:variant, element #11=w349:variant, element #12=w348:variant)  [unwired: 12 in]
          n133 = Index Array(array=w343) -> (element=w307:dbl)  [unwired: 1 in]
          n134 = Index Array(array=w338) -> (element=w302:dbl)  [unwired: 1 in]
          n135 = Index Array(array=w339) -> (element=w303:dbl)  [unwired: 1 in]
          n136 = Index Array(array=w337) -> (element=w301:dbl)  [unwired: 1 in]
          n137 = Index Array(array=w336) -> (element=w300:dbl)  [unwired: 1 in]
          n138 = Index Array(array=w342) -> (element=w306:dbl)  [unwired: 1 in]
          n139 = xnode "Database Variant To Data"("database variant"=w359, "error in (no error)"=w324, "type"=w311) -> ("data"=w335:i32, "error out"=w323:errorcluster)
          n140 = xnode "Database Variant To Data"("database variant"=w358, "error in (no error)"=w324, "type"=w310) -> ("data"=w299:dbl, "error out"=w298:errorcluster)
          n141 = xnode "Database Variant To Data"("database variant"=w357, "error in (no error)"=w324, "type"=w309) -> ("data"=w334:dbl, "error out"=w322:errorcluster)
          n142 = xnode "Database Variant To Data"("database variant"=w353, "error in (no error)"=w324, "type"=w305) -> ("data"=w333:dbl, "error out"=w321:errorcluster)
          n143 = xnode "Database Variant To Data"("database variant"=w356, "error in (no error)"=w324, "type"=w308) -> ("data"=w332:dbl, "error out"=w320:errorcluster)
          n144 = xnode "Database Variant To Data"("database variant"=w352, "error in (no error)"=w324, "type"=w304) -> ("data"=w330:dbl, "error out"=w319:errorcluster)
          n145 = xnode "Database Variant To Data"("database variant"=w355, "error in (no error)"=w324, "type"=w307) -> ("data"=w331:dbl, "error out"=w318:errorcluster)
          n146 = xnode "Database Variant To Data"("database variant"=w351, "error in (no error)"=w324, "type"=w302) -> ("data"=w328:dbl, "error out"=w317:errorcluster)
          n147 = xnode "Database Variant To Data"("database variant"=w349, "error in (no error)"=w324, "type"=w303) -> ("data"=w329:dbl, "error out"=w316:errorcluster)
          n148 = xnode "Database Variant To Data"("database variant"=w350, "error in (no error)"=w324, "type"=w301) -> ("data"=w327:dbl, "error out"=w315:errorcluster)
          n149 = xnode "Database Variant To Data"("database variant"=w348, "error in (no error)"=w324, "type"=w300) -> ("data"=w326:dbl, "error out"=w314:errorcluster)
          n150 = xnode "Database Variant To Data"("database variant"=w354, "error in (no error)"=w324, "type"=w306) -> ("data"=w325:dbl, "error out"=w313:errorcluster)
          n151 = Merge Errors(w323, w298, w322, w321, w320, w319, w318, w317, w316, w315, w314, w313) -> (w312:errorcluster)
        }
        n152 = Bundle By Name(cluster=w258, "Pelletron ID"=w271, "Integer Timestamp"=w270, "High Voltage"=w269, "Positive High Voltage Supply"=w267, "Negative High Voltage Supply"=w266, "Vaccuum Pressure"=w268, "Radiation"=w265, "Chain Current"=w264, "Column Current"=w263, "Lost Charge"=w262, "High Voltage Control"=w261, "Control Difference"=w260) -> (w259:T5)
      }
      event "Limits": Value Change {
        n153 = event-data() -> ("NewVal"=w748:T2)  [unwired: 1 in, 4 out]
        n154 = local write "Limits 2"(w748) -> ()
      }
      event "Limits 2": Value Change {
        n155 = event-data() -> ()  [unwired: 1 in, 5 out]
        n156 = local write "Limits"("Limits 2") -> ()
      }
      event "Y Minimum", "Y Maximum": Value Change {
        n157 = event-data() -> ()  [unwired: 1 in, 5 out]
        n158 = property on="XY Graph" class="XYGraph (strict)"(error in=w756, "ActYScl"="Active Y Scale", "YScale.Maximum"="Y Maximum", "YScale.Minimum"="Y Minimum", "YScale.ScaleFit"=u8 0 ("Y Scale.Scale Fit")) -> (error out=w755:errorcluster)  [unwired: 1 in, 1 out]
        n159 = local write "Y Autoscale"(FALSE ("Y Autoscale")) -> ()
      }
      event "X Minimum", "X Maximum": Value Change {
        n160 = event-data() -> ()  [unwired: 1 in, 5 out]
        n161 = property on="XY Graph" class="XYGraph (strict)"(error in=w766, "XScale.Maximum"="X Maximum", "XScale.Minimum"="X Minimum", "XScale.ScaleFit"=u8 0 ("X Scale.Scale Fit")) -> (error out=w765:errorcluster)  [unwired: 1 in, 1 out]
        n162 = local write "X Autoscale"(FALSE ("X Autoscale")) -> ()
      }
      event "Active Y Scale": Value Change {
        n163 = event-data() -> ("NewVal"=w773:u16)  [unwired: 1 in, 4 out]
        n164 = property on="XY Graph" class="XYGraph (strict)"("ActYScl"=w773) -> (error out=w772:errorcluster)  [unwired: 2 in, 1 out]
        n165 = property on="XY Graph" class="XYGraph (strict)"(error in=w772) -> ("YScale.Maximum"=w771:dbl, "YScale.Minimum"=w770:dbl)  [unwired: 1 in, 2 out]
        n166 = local write "Y Maximum"(w771) -> ()
        n167 = local write "Y Minimum"(w770) -> ()
      }
      event "Write": Value Change {
        n168 = event-data() -> ()  [unwired: 1 in, 5 out]
        n169 = property on="Pelletron Data" class="Tbl (strict)"() -> ("Column Headers[]"=w780:string[])  [unwired: 2 in, 2 out]
        n170 = local read "Pelletron Data"() -> (w778:string[][])
        n171 = for {
          tunnel: w780 -> [w789] mode=indexing
          tunnel: [w787] -> w779 mode=indexing
          n172 = call <vilib>:"Space Constant.vi"() -> ("String"=w788:string)
          n173 = Search and Replace String(input string=w789, search string="\n", replace string=w788) -> (result string=w787:string)  [unwired: 5 in, 3 out]
        }
        n174 = Build Array (concatenate)(w779, w778) -> (w777:string[][])
        n175 = call-poly <vilib>:"Write To Spreadsheet File.vi"("delimiter (\\t)"="," ("delimiter (\\t)"), "2D data"=w777, "file path (dialog if empty)"="Save Path") -> ()  [unwired: 5 in, 1 out]
        n176 = flat-sequence {
          frame #0 {
            n177 = Wait (ms)(milliseconds to wait=u32 100) -> ()  [unwired: 1 out]
          }
          frame #1 {
            n178 = local write "Write"(FALSE ("Write")) -> ()
          }
        }
      }
    }
  }
